vi "Reshape_Dots_To_Matrix1.vi"(4 "# cols":i32, 5 "# Gaps":i32, 6 "error IN":errorcluster, 7 "Starting Pos":i32[](array[numeric]), 8 "# rows":i32, 10 "Dot seq (in columns)":dbl[][](array[numeric])) -> (0 "error OUT":errorcluster, 3 "FR-TO-FR dot\nsequence":dbl[][](array[numeric]))   [LabVIEW 2013]
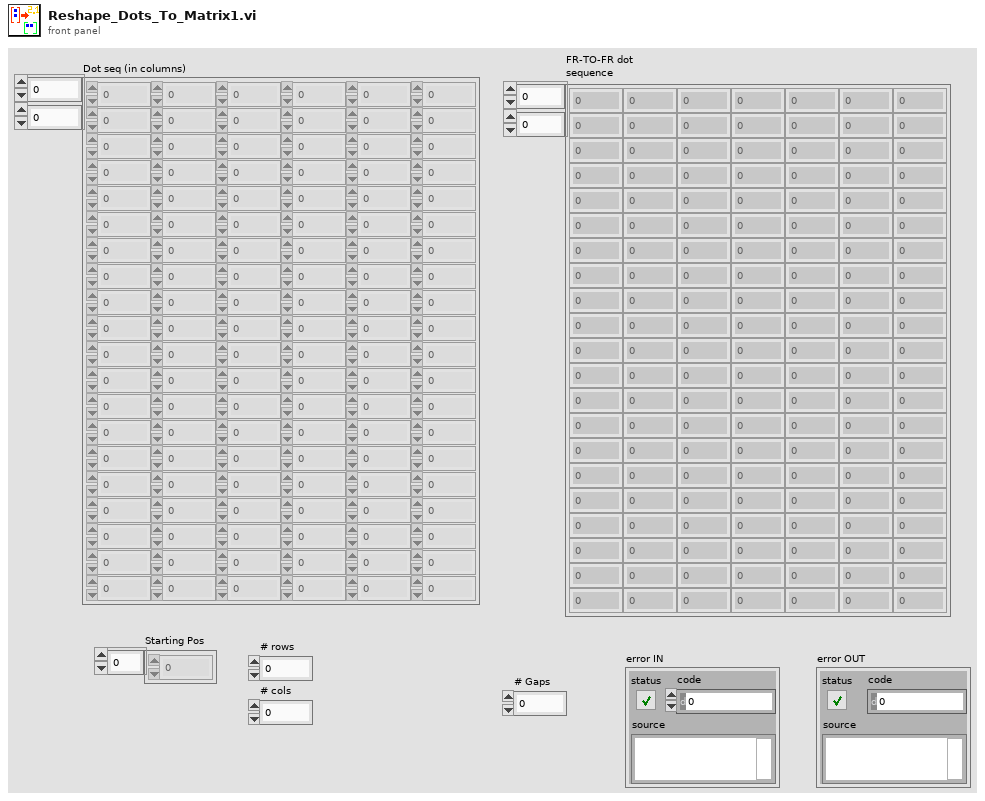
[diagram p1: front panel]
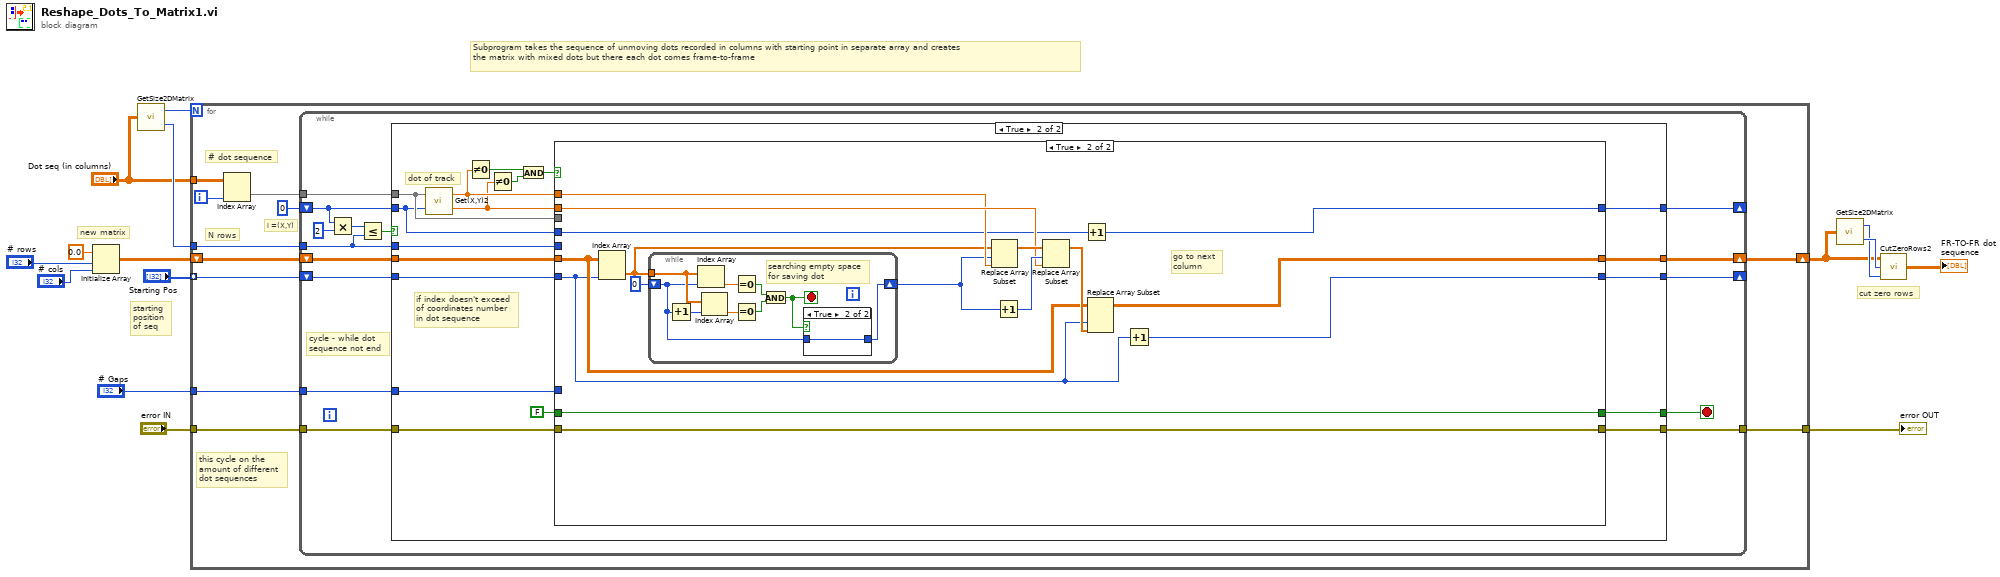
[diagram p0: block diagram]
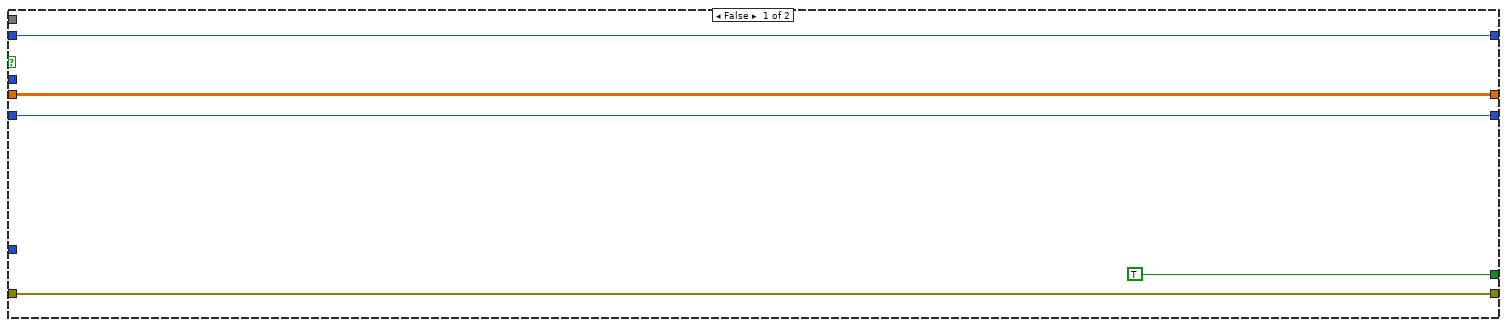
[diagram p2: hidden frame]
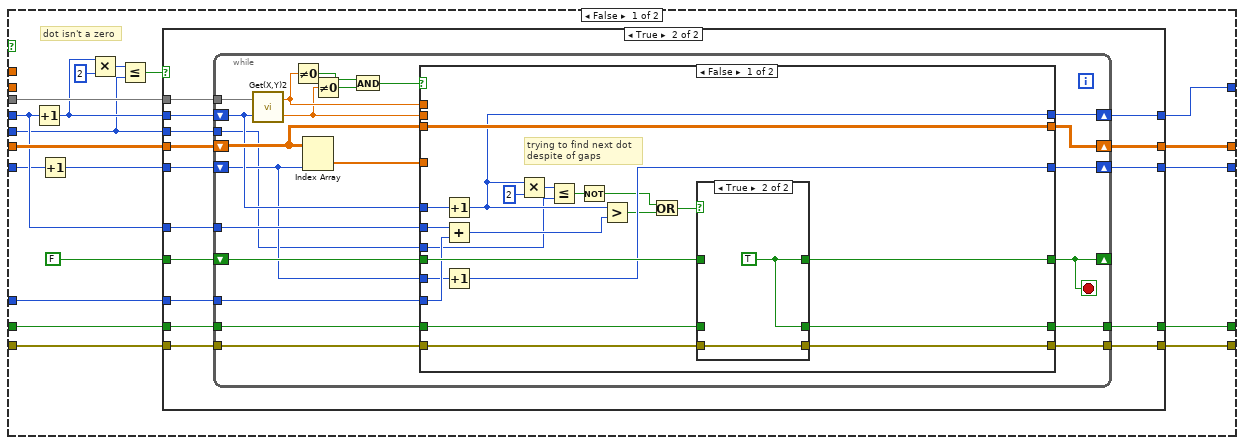
[diagram p3: hidden frame]
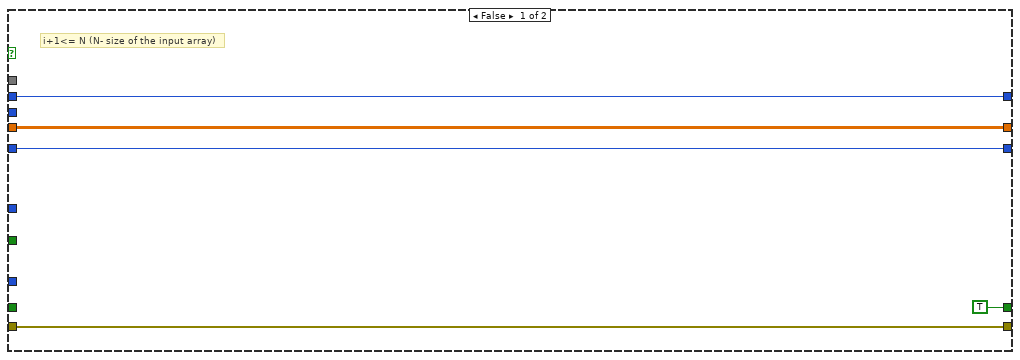
[diagram p4: hidden frame]
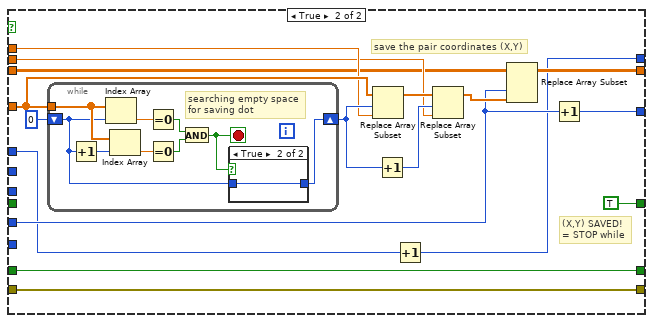
[diagram p6: hidden frame]
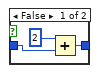
[diagram p7: hidden frame]
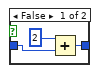
[diagram p8: hidden frame]
diagram:
  # "cut zero rows"
  # "starting \nposition\nof seq"
  # "Subprogram takes the sequence of unmoving dots recorded in columns with starting point in separate array and creates \nthe matrix with mixed dots but there each dot comes frame-to-frame"
  # "new matrix"
  n1 = Initialize Array(0.0 ("element"), "# rows", "# cols") -> (w11:dbl[][])
  n2 = call "GetSize2DMatrix.vi"("Array IN (2D)"="Dot seq (in columns)") -> ("# Cols"=w12:i32, "# Rows"=w8:i32)
  n3 = for {
    N: w12 -> [_]
    tunnel: "Dot seq (in columns)" -> [w26]
    shift-right: [w21] -> w3
    shift-left: w11 -> [w22]
    tunnel: "Starting Pos" -> [w23] mode=indexing
    tunnel: "# Gaps" -> [w19]
    tunnel: w8 -> [w18]
    tunnel: "error IN" -> [w17]
    tunnel: [w16] -> w4
    i -> [w25]
    # "i =(X,Y)"
    # "N rows"
    # "this cycle on the \namount of different\ndot sequences"
    # "# dot sequence"
    n4 = Index Array(array=w26, index (col)=w25) -> (element=w24:dbl[])  [unwired: 1 in]
    n5 = while {
      tunnel: w24 -> [w38]
      shift-right: [w40] -> w21
      shift-left: w22 -> [w37]
      shift-right: [w41] -> _
      shift-left: w23 -> [w36]
      shift-right: [w39] -> _
      shift-left: 0 -> [w31]
      tunnel: w19 -> [w35]
      tunnel: w18 -> [w28]
      tunnel: w17 -> [w33]
      tunnel: [w32] -> w16
      stop <- w34 stop-if-true
      # "cycle - while dot\nsequence not end"
      n6 = Multiply(x=w31, y=2) -> (x*y=w29:i32)
      n7 = Less Or Equal?(x=w29, y=w28) -> (x <= y?=w27:bool)
      n8 = case shown="True" w27 {
        tunnel: [w45 w62] -> w41
        tunnel: [w46 w61] -> w40
        tunnel: [w42 w60] -> w39
        tunnel: w38 -> [_ w57]
        tunnel: w31 -> [w42 w56]
        tunnel: w28 -> [_ w55]
        tunnel: w37 -> [w46 w54]
        tunnel: w36 -> [w45 w53]
        tunnel: w35 -> [_ w52]
        tunnel: [TRUE w49] -> w34
        tunnel: w33 -> [w43 w48]
        tunnel: [w43 w47] -> w32
        frame False {
        }
        frame True {
          # "if index doesn't exceed\nof coordinates number\nin dot sequence"
          # "dot of track"
          n9 = call "Get(X,Y)2.vi"("[IN] index of (X,Y)"=w56, "[IN] Array coordi\nnates (X,Y) in Frame"=w57) -> ("[OUT] Y"=w58:dbl, "[OUT] X"=w59:dbl)
          n10 = Not Equal To 0?(x=w59) -> (x != 0?=w64:bool)
          n11 = Not Equal To 0?(x=w58) -> (x != 0?=w63:bool)
          n12 = And(x=w64, y=w63) -> (x .and. y?=w51:bool)
          n13 = case shown="True" w51 {
            tunnel: w54 -> [w81 w186]
            tunnel: [w80 w195] -> w61
            tunnel: w58 -> [_ w193]
            tunnel: w59 -> [_ w192]
            tunnel: [w78 w191] -> w62
            tunnel: w56 -> [w73 w190]
            tunnel: w52 -> [w83 _]
            tunnel: [w79 w189] -> w60
            tunnel: w57 -> [w82 _]
            tunnel: w53 -> [w71 w185]
            tunnel: w55 -> [w66 _]
            tunnel: FALSE -> [w77 w183]
            tunnel: [w76 w183] -> w49
            tunnel: w48 -> [w75 w182]
            tunnel: [w74 w182] -> w47
            frame False {
              # "dot isn't a zero"
              n14 = Increment(x=w73) -> (x+1=w67:i32)
              n15 = Increment(x=w71) -> (x+1=w70:i32)
              n16 = Multiply(x=w67, y=2) -> (x*y=w68:i32)
              n17 = Less Or Equal?(x=w68, y=w66) -> (x <= y?=w65:bool)
              n18 = case shown="True" w65 {
                tunnel: w83 -> [_ w103]
                tunnel: w82 -> [_ w102]
                tunnel: w67 -> [w86 w101]
                tunnel: w81 -> [w84 w100]
                tunnel: w66 -> [_ w99]
                tunnel: [w84 w98] -> w80
                tunnel: [w86 w97] -> w79
                tunnel: [w85 w96] -> w78
                tunnel: w77 -> [_ w95]
                tunnel: [TRUE w94] -> w76
                tunnel: w75 -> [w88 w93]
                tunnel: [w88 w92] -> w74
                tunnel: w73 -> [_ w91]
                tunnel: FALSE -> [_ w90]
                tunnel: w70 -> [w85 w89]
                frame False {
                  # "i+1<= N (N- size of the input array)"
                }
                frame True {
                  n19 = while {
                    shift-right: [w114] -> w97
                    shift-left: w101 -> [w117]
                    tunnel: w103 -> [w115]
                    tunnel: w102 -> [w125]
                    shift-right: [w116] -> w98
                    shift-left: w100 -> [w119]
                    tunnel: w99 -> [w104]
                    shift-right: [w118] -> w96
                    shift-left: w89 -> [w105]
                    tunnel: w95 -> [w113]
                    tunnel: [w112] -> w94
                    tunnel: w93 -> [w111]
                    tunnel: [w110] -> w92
                    tunnel: w91 -> [w109]
                    shift-right: [w108] -> _
                    shift-left: w90 -> [w107]
                    stop <- w108 stop-if-true
                    n20 = call "Get(X,Y)2.vi"("[IN] index of (X,Y)"=w117, "[IN] Array coordi\nnates (X,Y) in Frame"=w125) -> ("[OUT] Y"=w121:dbl, "[OUT] X"=w122:dbl)
                    n21 = Not Equal To 0?(x=w122) -> (x != 0?=w124:bool)
                    n22 = Index Array(array=w119, index (col)=w105) -> (element=w120:dbl[])  [unwired: 1 in]
                    n23 = Not Equal To 0?(x=w121) -> (x != 0?=w123:bool)
                    n24 = And(x=w124, y=w123) -> (x .and. y?=w106:bool)
                    n25 = case shown="False" w106 {
                      tunnel: w122 -> [_ w163]
                      tunnel: w121 -> [_ w162]
                      tunnel: w107 -> [w145 _]
                      tunnel: w120 -> [_ w164]
                      tunnel: w119 -> [w146 w161]
                      tunnel: w105 -> [w136 w159]
                      tunnel: [w135 w158] -> w118
                      tunnel: w117 -> [w139 w156]
                      tunnel: [w146 w157] -> w116
                      tunnel: w115 -> [w137 _]
                      tunnel: [w144 TRUE] -> w108
                      tunnel: [w131 w155] -> w114
                      tunnel: w113 -> [w143 w153]
                      tunnel: [w142 w153] -> w112
                      tunnel: w111 -> [w141 w152]
                      tunnel: [w140 w152] -> w110
                      tunnel: w109 -> [w138 _]
                      tunnel: w104 -> [w130 _]
                      frame False {
                        # "trying to find next dot\ndespite of gaps"
                        n26 = Increment(x=w139) -> (x+1=w131:i32)
                        n27 = Add(x=w138, y=w137) -> (x+y=w134:i32)
                        n28 = Increment(x=w136) -> (x+1=w135:i32)
                        n29 = Multiply(x=w131, y=2) -> (x*y=w132:i32)
                        n30 = Less Or Equal?(x=w132, y=w130) -> (x <= y?=w129:bool)
                        n31 = Not(x=w129) -> (.not. x?=w127:bool)
                        n32 = Greater?(x=w131, y=w134) -> (0:w128:bool)
                        n33 = Or(x=w127, y=w128) -> (x .or. y?=w126:bool)
                        n34 = case shown="True" w126 {
                          tunnel: w145 -> [w149 _]
                          tunnel: [w149 w151] -> w144
                          tunnel: w143 -> [w148 _]
                          tunnel: [w148 w151] -> w142
                          tunnel: w141 -> [w147 w150]
                          tunnel: [w147 w150] -> w140
                          frame False {
                          }
                          frame True {
                            w151 = TRUE
                          }
                        }
                      }
                      frame True {
                        # "(X,Y) SAVED!\n= STOP while"
                        # "save the pair coordinates (X,Y)"
                        n35 = while {
                          tunnel: w164 -> [w175]
                          shift-right: [w169] -> w165
                          shift-left: 0 -> [w170]
                          stop <- w171 stop-if-true
                          # "searching empty space\nfor saving dot"
                          n36 = Increment(x=w170) -> (x+1=w176:i32)
                          n37 = Index Array(array=w175, index=w170) -> (element=w177:dbl)
                          n38 = Index Array(array=w175, index=w176) -> (element=w174:dbl)
                          n39 = Equal To 0?(x=w177) -> (x = 0?=w173:bool)
                          n40 = Equal To 0?(x=w174) -> (x = 0?=w172:bool)
                          n41 = And(x=w173, y=w172) -> (x .and. y?=w171:bool)
                          n42 = case shown="True" w171 {
                            tunnel: w170 -> [w179 w181]
                            tunnel: [w180 w181] -> w169
                            frame False {
                              n43 = Add(x=2, y=w179) -> (x+y=w180:i32)
                            }
                            frame True {
                            }
                          }
                        }
                        n44 = Replace Array Subset(array=w164, new element=w163, index=w165) -> (w167:dbl[])
                        n45 = Increment(x=w165) -> (x+1=w166:i32)
                        n46 = Increment(x=w156) -> (x+1=w155:i32)
                        n47 = Replace Array Subset(array=w167, new element=w162, index=w166) -> (w160:dbl[])
                        n48 = Replace Array Subset(array=w161, new element=w160, index (col)=w159) -> (w157:dbl[][])  [unwired: 1 in]
                        n49 = Increment(x=w159) -> (x+1=w158:i32)
                      }
                    }
                  }
                }
              }
            }
            frame True {
              # "go to next \ncolumn"
              n50 = Index Array(array=w186, index (col)=w185) -> (element=w184:dbl[])  [unwired: 1 in]
              n51 = while {
                tunnel: w184 -> [w204]
                shift-right: [w198] -> w187
                shift-left: 0 -> [w199]
                stop <- w200 stop-if-true
                # "searching empty space\nfor saving dot"
                n52 = Increment(x=w199) -> (x+1=w205:i32)
                n53 = Index Array(array=w204, index=w199) -> (element=w206:dbl)
                n54 = Index Array(array=w204, index=w205) -> (element=w203:dbl)
                n55 = Equal To 0?(x=w206) -> (x = 0?=w202:bool)
                n56 = Equal To 0?(x=w203) -> (x = 0?=w201:bool)
                n57 = And(x=w202, y=w201) -> (x .and. y?=w200:bool)
                n58 = case shown="True" w200 {
                  tunnel: w199 -> [w208 w210]
                  tunnel: [w209 w210] -> w198
                  frame False {
                    n59 = Add(x=2, y=w208) -> (x+y=w209:i32)
                  }
                  frame True {
                  }
                }
              }
              n60 = Replace Array Subset(array=w184, new element=w192, index=w187) -> (w197:dbl[])
              n61 = Increment(x=w187) -> (x+1=w196:i32)
              n62 = Replace Array Subset(array=w197, new element=w193, index=w196) -> (w194:dbl[])
              n63 = Increment(x=w190) -> (x+1=w189:i32)
              n64 = Replace Array Subset(array=w186, new element=w194, index (col)=w185) -> (w195:dbl[][])  [unwired: 1 in]
              n65 = Increment(x=w185) -> (x+1=w191:i32)
            }
          }
        }
      }
    }
  }
  "error OUT" <- w4
  n66 = call "GetSize2DMatrix.vi"("Array IN (2D)"=w3) -> ("# Cols"=w6:i32, "# Rows"=w7:i32)
  n67 = call "CutZeroRows2.vi"("# Cols"=w6, "# Rows"=w7, "Array IN"=w3) -> ("Array OUT"=→"FR-TO-FR dot\nsequence":dbl[][])
